vi "SendLogMsg.vi"(8 "error in (no error)":errorcluster, 10 "LogMsg":cluster{"Cmd":string, "Data":variant}, 11 "Queue In":refnum<queue>) -> (0 "error out":errorcluster, 3 "Queue Out":refnum<queue>)   [LabVIEW 2016, in "Log4Lv.lvlib"]
doc: "Use this template to build a VI to use as a subVI."
uses:
  Log4Lv.lvlib
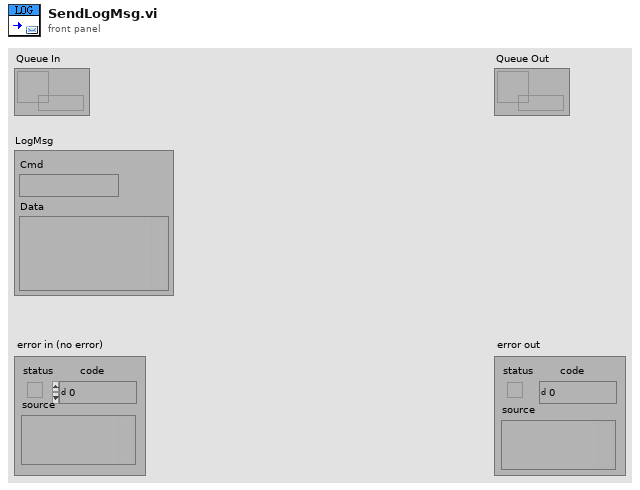
[diagram p1: front panel]
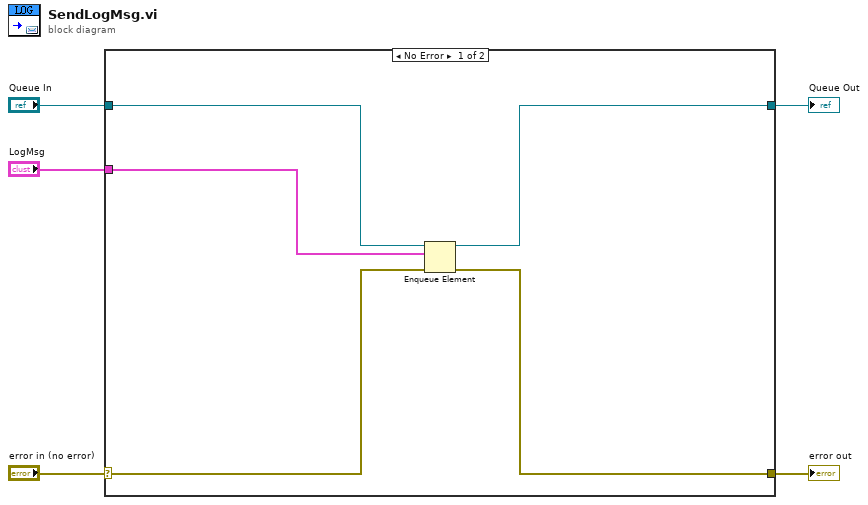
[diagram p0: block diagram]
diagram:
  n1 = case shown="No Error" "error in (no error)" {
    selector: "error in (no error)" -> [w8 w12]
    tunnel: [w7 w12] -> w4
    tunnel: [w9 w11] -> w3
    tunnel: "Queue In" -> [w10 w11]
    tunnel: "LogMsg" -> [w6 _]
    frame No Error {
      n2 = Enqueue Element(queue=w10, element=w6, error in (no error)=w8) -> (queue out=w9:refnum<queue>, error out=w7:errorcluster)  [unwired: 1 in, 1 out]
    }
    frame Error {
    }
  }
  "error out" <- w4
  "Queue Out" <- w3
